vi "Variant to Tree.vi"(10 "Variant":variant) -> (2 "Variant Tree":variant)   [LabVIEW 2013, in "OpenVariant.lvlib"]
doc: "This VI takes a default value as the input and replaces it recursively (cluster, array) with values found in key value pair arrays."
uses:
  OpenVariant.lvlib
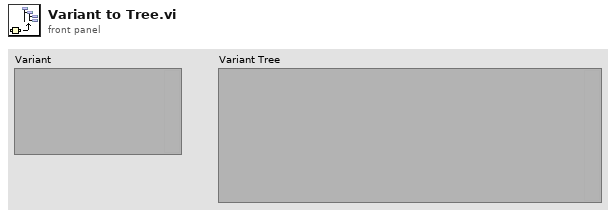
[diagram p1: front panel]
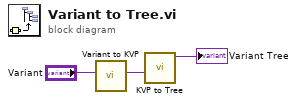
[diagram p0: block diagram]
diagram:
  n1 = call "Variant to KVP.vi"("Variant"="Variant") -> ("KVP Dictionary"=w2:variant)  [unwired: 10 in]
  n2 = call "KVP to Tree.vi"("KVP"=w2) -> ("Variant Tree"=→"Variant Tree":variant)  [unwired: 10 in]
